vi "MGI 3D Target 3D Camera.vi"(8 "error in (no error)":errorcluster, 10 "3D Target":cluster{"X":sgl, "Y":sgl, "Z":sgl}, 11 "SceneGraphDisplay in":refnum<vi>) -> (0 "error out":errorcluster, 3 "SceneGraphDisplay out":refnum<vi>)   [LabVIEW 2020]
doc: "Aim the 3D camera at a target specified in model space while maintaining orientation and zoom. Z-up orientation is assumed.\n\nAuthored by David A. Moore\nsupport@mooregoodideas.com\nwww.mooregoodideas.com\n\nCopyright (c) 2012, Moore Good Ideas, Inc.\n\nAll rights reserved.\n\nRedistribution and use in source and binary forms, with or without modification, are permitted provided that the following conditions are met:\n\n * Redistributions of source code must retain the above copyright notice, this list of conditions and the following disclaimer.\n * Redistributions in binary form must reproduce the above copyright notice, this list of conditions and the following disclaimer in the documentation and/or other materials provided with the distribution.\n * Neither the name of Moore Good Ideas, Inc. nor the names of its contributors may be used to endorse or promote products derived from this software without specific prior written permission.\n\nTHIS SOFTWARE IS PROVIDED BY THE COPYRIGHT HOLDERS AND CONTRIBUTORS \"AS IS\" AND ANY EXPRESS OR IMPLIED WARRANTIES, INCLUDING, BUT NOT LIMITED TO, THE IMPLIED WARRANTIES OF MERCHANTABILITY AND FITNESS FOR A PARTICULAR PURPOSE ARE DISCLAIMED. IN NO EVENT SHALL THE COPYRIGHT OWNER OR CONTRIBUTORS BE LIABLE FOR ANY DIRECT, INDIRECT, INCIDENTAL, SPECIAL, EXEMPLARY, OR CONSEQUENTIAL DAMAGES (INCLUDING, BUT NOT LIMITED TO, PROCUREMENT OF SUBSTITUTE GOODS OR SERVICES; LOSS OF USE, DATA, OR PROFITS; OR BUSINESS INTERRUPTION) HOWEVER CAUSED AND ON ANY THEORY OF LIABILITY, WHETHER IN CONTRACT, STRICT LIABILITY, OR TORT (INCLUDING NEGLIGENCE OR OTHERWISE) ARISING IN ANY WAY OUT OF THE USE OF THIS SOFTWARE, EVEN IF ADVISED OF THE POSSIBILITY OF SUCH DAMAGE."
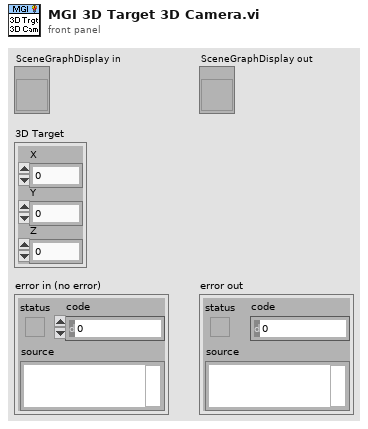
[diagram p1: front panel]
types:
  T1 = cluster{"ModelView Matrix[0]":sgl, "ModelView Matrix[1]":sgl, "ModelView Matrix[2]":sgl}
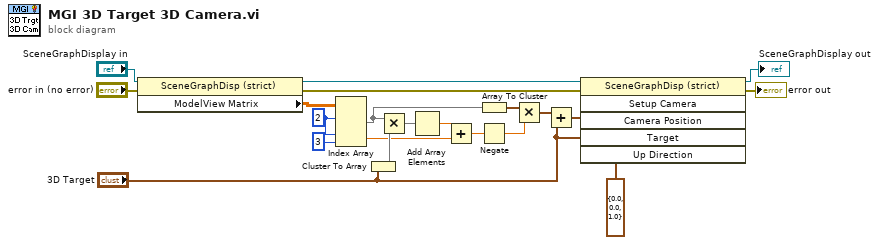
[diagram p0: block diagram]
diagram:
  w3 = 2 ("index (row)")
  n1 = property on="Property Node" class="SceneGraphDisp (strict)"(reference="SceneGraphDisplay in", error in="error in (no error)") -> (reference out=w18:refnum<vi>, error out=w20:errorcluster, "ModelView Matrix"=w17:sgl[][])
  n2 = Index Array(array=w17, index (row) #1=w3, index (row) #2=w3, index (col) #2=3 ("disabled index (col)")) -> (element #1=w12:sgl[], element #2=w5:sgl)  [unwired: 1 in]
  n3 = Cluster To Array(cluster="3D Target") -> (array=w11:sgl[])
  n4 = Multiply(x=w12, y=w11) -> (x*y=w13:sgl[])
  n5 = Add Array Elements(numeric array=w13) -> (sum=w14:sgl)
  n6 = Add(x=w14, y=w5) -> (x+y=w6:sgl)
  n7 = Array To Cluster(array=w12) -> (cluster=w7:T1)
  n8 = Negate(x=w6) -> (-x=w15:sgl)
  n9 = Multiply(x=w7, y=w15) -> (x*y=w8:T1)
  n10 = Add(x=w8, y="3D Target") -> (x+y=w9:cluster{sgl, sgl, sgl})
  n11 = invoke class="SceneGraphDisp (strict)" method="Setup Camera"(reference=w18, error in=w20, "Camera Position"=w9, "Target"="3D Target", "Up Direction"=cluster{"X":sgl, "Y":sgl, "Z":sgl} {"X"=0.0, "Y"=0.0, "Z"=1.0}) -> (reference out=→"SceneGraphDisplay out":refnum<vi>, error out=→"error out":errorcluster)  [unwired: 1 in, 4 out]
